vi "SetTopLevelInLLB.vi"(5 "Files Generated by Build":path[](array[path]), 6 "Top Level/Always Included VIs":path[](array[path]), 7 "Destination Path":path, 8 "error in (no error)":errorcluster, 9 "Target Name":string, 10 "Build Specification Name":string, 11 "Project Path":path) -> (0 "error out":errorcluster)   [LabVIEW 2014]
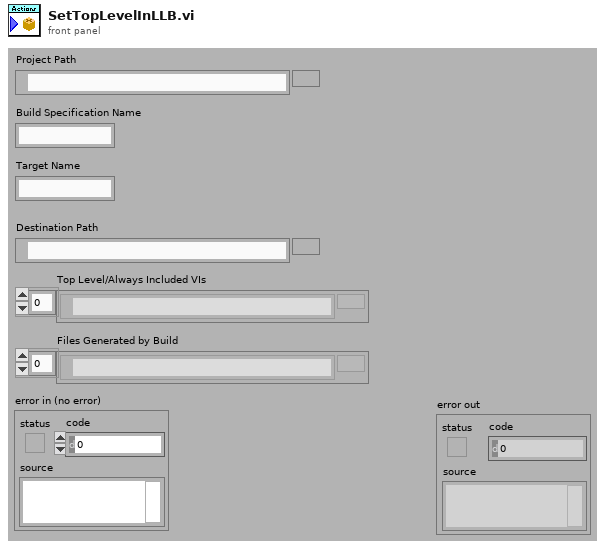
[diagram p1: front panel]
types:
  T1 = typedef "Librarian File Info Out.ctl" = cluster{"creation date":u32, "last mod date":u32, "type":string, "creator":string, "LV version":i32, "size":i32, "top level":bool}
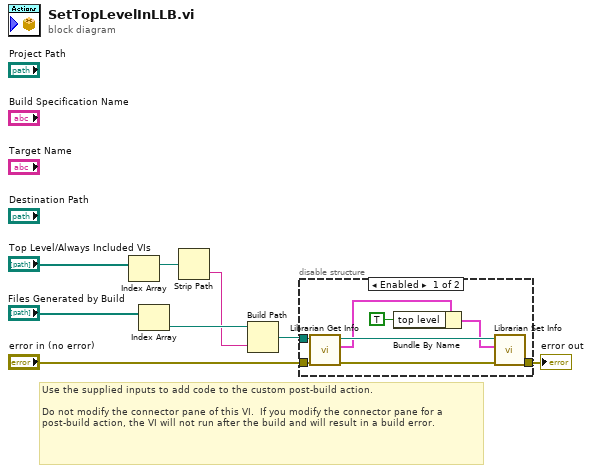
[diagram p0: block diagram]
diagram:
  # "Use the supplied inputs to add code to the custom post-build action.\n\nDo not modify the connector pane of this VI.  If you modify the connector pane for a post-build action, the VI will not run after the build and will result in a build error."
  n1 = Index Array(array="Top Level/Always Included VIs") -> (element=w5:path)  [unwired: 1 in]
  n2 = Index Array(array="Files Generated by Build") -> (element=w3:path)  [unwired: 1 in]
  n3 = Strip Path(path=w5) -> (name=w1:string)  [unwired: 1 out]
  n4 = Build Path(base path=w3, name or relative path=w1) -> (appended path=w2:path)
  n5 = disable-structure shown="Enabled" {
    disable-tunnel: "error in (no error)" -> [w16 w17]
    disable-tunnel: [w15 w17] -> w7
    disable-tunnel: w2 -> [w12 _]
    frame Enabled {
      n6 = call <vilib>:"Librarian Get Info.vi"("error in (no error)"=w16, "path"=w12) -> ("error out"=w14:errorcluster, "file information"=w11:T1, "dup path"=w13:path)  [unwired: 7 in]
      n7 = Bundle By Name(cluster=w11, "top level"=TRUE) -> (w9:T1)
      n8 = call <vilib>:"Librarian Set Info.vi"("error in (no error)"=w14, "file information"=w9, "path"=w13) -> ("error out"=w15:errorcluster)  [unwired: 7 in, 1 out]
    }
    frame Disabled {
    }
  }
  "error out" <- w7
